vi "Build XY Plot Histogram (Core).vi"(4 "Bin Size (Dialog)":dbl=nan, 5 "Align Histogram Bin":bool, 6 "Plot Index":i32, 7 "Max Number of Bins":i32, 8 "error in (no error)":errorcluster, 9 "Data Axis (Y: F)":bool, 10 "Mouse Click Coords":T1, 11 "XYGraph in":T2) -> (0 "error out":errorcluster, 1 "Message":string, 3 "Data Statistics":dbl[](array[numeric]))   [LabVIEW 2019, in "Histogram Window.lvlib"]
uses:
  Histogram Window.lvlib
  Graphs/XY Graph/XY Graph Refnum.ctl
  <vilib>/Utility/miscctls.llb/LVPoint32TypeDef.ctl
  Linear Histogram Options.ctl
  Histogram Bin Position.ctl
  Plot Histogram.ctl
  Graphs/Plot Style 3.ctl
  Histogram Window Q Element v2.ctl
  Histogram Window Q Action v2.ctl
  Data Statistics.ctl
  48084c95-8393-4bd0-bb26-e53c6117abf8.vi/ae578a56-f3ce-4ec2-8f3b-219cc1dae63b.vi
  <vilib>/Analysis/NI_AALBase.lvlib
  <vilib>/Analysis/NI_AALPro.lvlib
  Graphs/XY Graph/XY Graph Add-Ons.lvlib
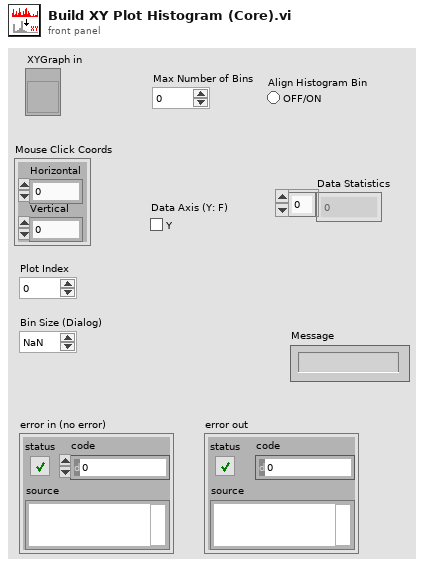
[diagram p1: front panel]
types:
  T1 = typedef "LVPoint32TypeDef.ctl" = cluster{"Horizontal":i32, "Vertical":i32}
  T2 = typedef "XY Graph Add-Ons.lvlib/XY Graph Refnum.ctl" = refnum<vi>
  T3 = typedef "Plot Style 3.ctl" = cluster{"Plot Style":enum16{"unchanged", "Line", "Symbol", "Line + Symbol", "Histogram", "Histogram + Symbol"}, "Histogram Type":enum16{"unchanged", "Left Bound", "Center", "Right Bound"}, "Line Tickness":enum16{"unchanged", "Thin", "1 pixel", "2 pixel", "3 pixel", "4 pixel", "5 pixel"}, "Line Style":enum16{"unchanged", "Plain", "Long Dash", "Short Dash", "Long-Short Dash", "Long-Short-Short Dash"}, "Point Style":enum16{"unchanged", "None", "Empty Circle", "Filled Circle", "Thick Circle", "Dotted Circle", "Empty Square", "Filled Square", "Thick Square", "Dotted Square", "Small Filled Square", "Dot", "Cross", "Tiny Cross", "Large X", "Small x", "Diamond", "Small Empty Square"}, "Line Color":u32, "Point Color":u32, "Anti-aliased":bool, "Line Color Chooser":enum16{"unchanged", "Color Box", "Color List"}, "Point Color Chooser":enum16{"unchanged", "Color Box", "Color List"}, "Line Color List":string, "Point Color List":string}
  T4 = typedef "Histogram Window.lvlib/Data Statistics.ctl" = cluster{"mean":dbl, "standard deviation":dbl, "variance":dbl, "rms value":dbl, "median":dbl, "mode":dbl, "max Value":dbl, "min Value":dbl, "# elements  ":dbl}
  T5 = typedef "Histogram Window.lvlib/Histogram Window Q Element v2.ctl" = cluster{"Histogram Window Q Action":T6, "Data":variant}
  T6 = typedef "Histogram Window.lvlib/Histogram Window Q Action v2.ctl" = enum16{"Idle", "Initialization", "Generic XY Graph Event", "Add Histogram", "Delete Plot", "Delete Selected Plots", "Clear Graph", "Change Bin Size", "Invert Histogram", "Update Graph", "Plot Fit", "Export XYGraph to Notebook", "Quit"}
  T7 = typedef "Histogram Window.lvlib/Plot Histogram.ctl" = cluster{"Plot Name":string, "Histogram":cluster{"Axis":dbl[], "Histogram":dbl[]}, "Plot Style":T3}
  T8 = typedef "Linear Histogram Options.ctl" = cluster{"Bin Size":dbl, "Min Value":dbl, "Max Value":dbl, "Filter NaN & Infinite Values":bool, "Frequency Plot":bool, "Align Bins":bool, "Bin Location":T9, "Project Outside Values":bool, "Max Histogram Size":i32}
  T9 = typedef "Histogram Bin Position.ctl" = enum16{"Left", "Center", "Right"}
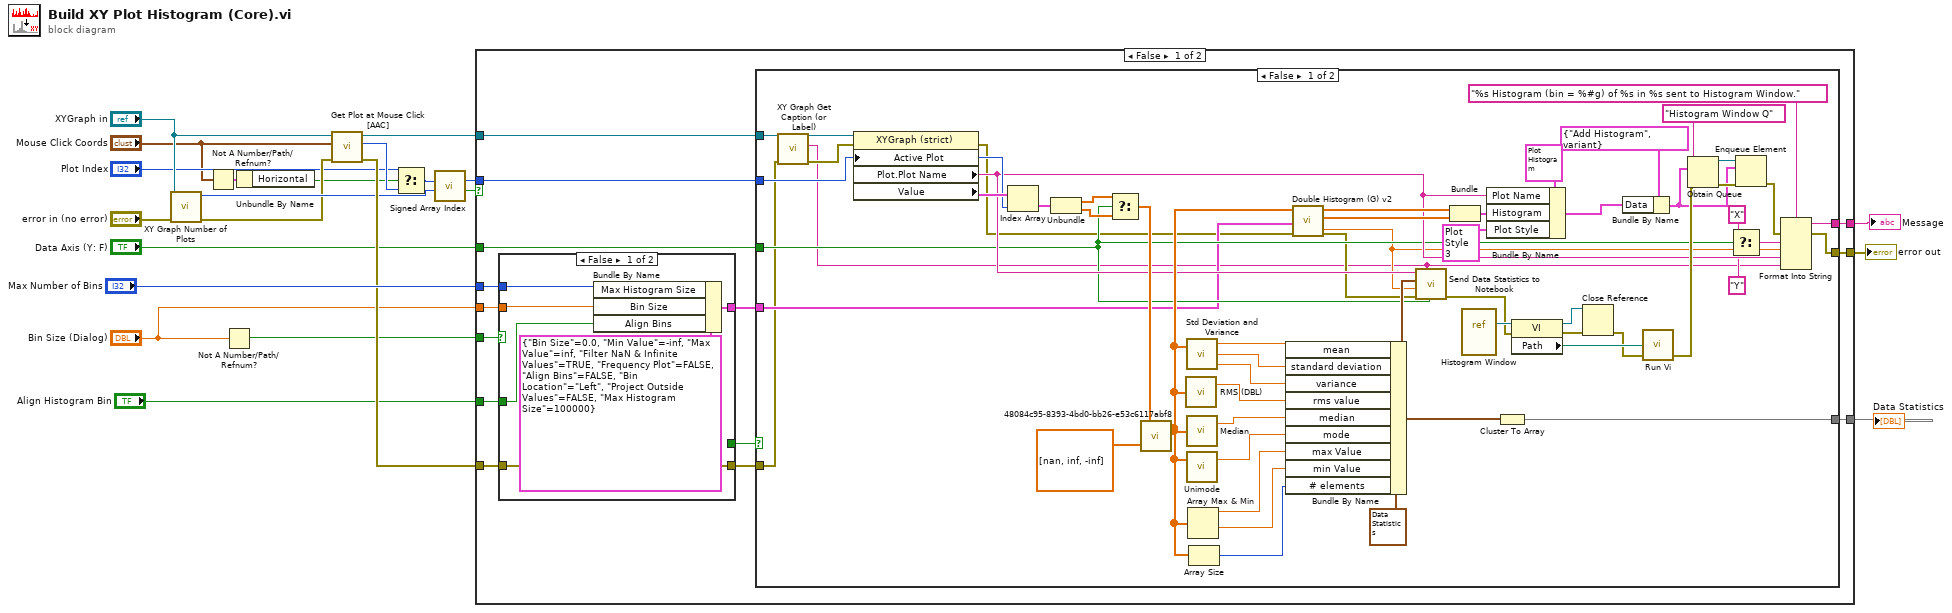
[diagram p0: block diagram]
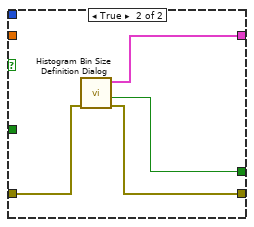
[diagram p3: hidden frame]
diagram:
  n1 = call "XY Graph Number of Plots.vi"("Error In"="error in (no error)", "XYGraph in"="XYGraph in") -> ("Error Out"=w15:errorcluster, "# Plots"=w18:i32)  [unwired: 8 in]
  n2 = Not A Number/Path/Refnum?(number/path/refnum="Mouse Click Coords") -> (NaN/Path/Refnum?=w7:cluster{"Horizontal":bool, "Vertical":bool})
  n3 = Not A Number/Path/Refnum?(number/path/refnum="Bin Size (Dialog)") -> (NaN/Path/Refnum?=w11:bool)
  n4 = Unbundle By Name(w7) -> ("Horizontal"=w8:bool)
  n5 = call "Get Plot at Mouse Click [AAC].vi"("error in (no error)"=w15, "Mouse Click Coordinates"="Mouse Click Coords", "XYGraph Ref"="XYGraph in") -> ("error out"=w20:errorcluster, "Plot at Coordinates"=w10:i32, "XYGraph Ref"=w4:T2)  [unwired: 2 in, 4 out]
  n6 = Select(t="Plot Index", s=w8, f=w10) -> (s? t:f=w16:i32)
  n7 = call "Signed Array Index.vi"("Array Size"=w18, "Array Index in"=w16) -> ("Out of Range?"=w19:bool, "Array Index out"=w17:i32)  [unwired: 8 in]
  n8 = case shown="False" w19 {
    tunnel: [w35 w104] -> w22
    tunnel: w4 -> [w36 _]
    tunnel: "Max Number of Bins" -> [w25 _]
    tunnel: w20 -> [w31 w104]
    tunnel: [w30 _] -> w5
    tunnel: w11 -> [w29 _]
    tunnel: "Bin Size (Dialog)" -> [w28 _]
    tunnel: w17 -> [w34 _]
    tunnel: "Data Axis (Y: F)" -> [w27 _]
    tunnel: [w26 _] -> w2
    tunnel: "Align Histogram Bin" -> [w23 _]
    frame False {
      n9 = case shown="False" w29 {
        tunnel: [_ w101] -> w33
        tunnel: [w99 w103] -> w32
        tunnel: w31 -> [w99 w102]
        tunnel: w28 -> [w97 _]
        tunnel: w25 -> [w98 _]
        tunnel: [w95 w100] -> w24
        tunnel: w23 -> [w94 _]
        frame False {
          n10 = Bundle By Name(cluster=T8 {"Bin Size"=0.0, "Min Value"=-inf, "Max Value"=inf, "Filter NaN & Infinite Values"=TRUE, "Frequency Plot"=FALSE, "Align Bins"=FALSE, "Bin Location"=enum."Left", "Project Outside Values"=FALSE, "Max Histogram Size"=100000} ("input cluster"), "Max Histogram Size"=w98, "Bin Size"=w97, "Align Bins"=w94) -> (w95:T8)
        }
        frame True {
          n11 = call "Histogram Bin Size Definition Dialog.vi"("error in (no error)"=w102) -> ("error out"=w103:errorcluster, "Cancelled?"=w101:bool, "Histogram Options"=w100:T8)  [unwired: 8 in]
        }
      }
      n12 = case shown="False" w33 {
        tunnel: w36 -> [w41 _]
        tunnel: [w58 w93] -> w35
        tunnel: w34 -> [w71 _]
        tunnel: w32 -> [w38 w93]
        tunnel: [w65 _] -> w30
        tunnel: w27 -> [w52 _]
        tunnel: [w57 _] -> w26
        tunnel: w24 -> [w44 _]
        frame False {
          n13 = call "XY Graph Get Caption (or Label).vi"("error in (no error)"=w38, "XYGraph in"=w41) -> ("error out"=w39:errorcluster, "Caption (or Label) Text"=w37:string, "XYGraph out"=w40:T2)  [unwired: 7 in]
          n14 = property class="XYGraph (strict)"(reference=w40, error in=w39, "Active Plot"=w71) -> (error out=w43:errorcluster, "Plot.Plot Name"=w55:string, "Value"=w84:cluster{"X Array":dbl[], "Y Array":dbl[]}[])  [unwired: 1 out]
          n15 = Index Array(array=w84, index=w71) -> (element=w83:cluster{"X Array":dbl[], "Y Array":dbl[]})
          n16 = Unbundle(w83) -> ("X Array"=w62:dbl[], "Y Array"=w61:dbl[])
          n17 = Select(t=w62, s=w52, f=w61) -> (s? t:f=w60:dbl[])
          n18 = call "48084c95-8393-4bd0-bb26-e53c6117abf8.vi"("Element(s) to Remove"=dbl[] [nan, inf, -inf], "Input Array"=w60) -> ("Output Array"=w63:dbl[])  [unwired: 1 out]
          n19 = call <vilib>:"RMS (DBL).vi"("X"=w63) -> ("rms value"=w77:dbl)  [unwired: 1 out]
          n20 = call <vilib>:"Std Deviation and Variance.vi"("X"=w63) -> ("mean"=w80:dbl, "standard deviation"=w79:dbl, "variance"=w78:dbl)  [unwired: 1 in]
          n21 = call <vilib>:"Median.vi"("X"=w63) -> ("median"=w76:dbl)  [unwired: 1 out]
          n22 = call <vilib>:"Unimode.vi"("X"=w63) -> ("mode"=w75:dbl)  [unwired: 1 in, 1 out]
          n23 = Array Max & Min(array=w63) -> (max value=w74:dbl, min value=w73:dbl)  [unwired: 2 out]
          n24 = Array Size(array=w63) -> (size(s)=w72:i32)
          n25 = Bundle By Name(cluster=T4 {"mean"=0.0, "standard deviation"=0.0, "variance"=0.0, "rms value"=0.0, "median"=0.0, "mode"=0.0, "max Value"=0.0, "min Value"=0.0, "# elements  "=0.0} ("Data Statistics"), "mean"=w80, "standard deviation"=w79, "variance"=w78, "rms value"=w77, "median"=w76, "mode"=w75, "max Value"=w74, "min Value"=w73, "# elements"=w72) -> (w66:T4)
          n26 = call "Double Histogram (G) v2.vi"("Error In"=w43, "Histogram Options"=w44, "Array"=w63) -> ("Error Out"=w42:errorcluster, "Histogram"=w86:dbl[], "Axis"=w85:dbl[], "Actual Bin Size"=w45:dbl)  [unwired: 4 in, 1 out]
          n27 = call "Send Data Statistics to Notebook.vi"("Data Axis (Y: F)"=w52, "Graph Caption"=w37, "Error In"=w42, "Bin"=w45, "Data Statistics"=w66, "Plot Name"=w55) -> ("Error Out"=w67:errorcluster)  [unwired: 5 in]
          n28 = Bundle("Axis"=w85, "Histogram"=w86) -> (w91:cluster{"Axis":dbl[], "Histogram":dbl[]})  [unwired: 1 in]
          n29 = vi-ref "Histogram Window.vi"() -> (w70:refnum<vi>)
          n30 = Bundle By Name(cluster=T7 {"Plot Name"="", "Histogram"={"Axis"=[], "Histogram"=[]}, "Plot Style"={"Plot Style"=enum."Histogram + Symbol", "Histogram Type"=enum."Right Bound", "Line Tickness"=enum."unchanged", "Line Style"=enum."unchanged", "Point Style"=enum."unchanged", "Line Color"=0, "Point Color"=0, "Anti-aliased"=FALSE, "Line Color Chooser"=enum."unchanged", "Point Color Chooser"=enum."unchanged", "Line Color List"="", "Point Color List"=""}} ("output cluster"), "Plot Name"=w55, "Histogram"=w91, "Plot Style"=T3 {"Plot Style"=enum."Histogram", "Histogram Type"=enum."Left Bound", "Line Tickness"=enum."1 pixel", "Line Style"=enum."Plain", "Point Style"=enum."None", "Line Color"=0, "Point Color"=0, "Anti-aliased"=TRUE, "Line Color Chooser"=enum."Color Box", "Point Color Chooser"=enum."unchanged", "Line Color List"="", "Point Color List"=""}) -> (w87:T7)
          n31 = Cluster To Array(cluster=w66) -> (array=w65:dbl[])
          n32 = property class="VI"(reference=w70, error in=w67) -> (reference out=w69:refnum<vi>, error out=w47:errorcluster, "Path"=w68:path)
          n33 = Close Reference(reference=w69, error in (no error)=w47) -> (error out=w46:errorcluster)
          n34 = Bundle By Name(cluster=T5 {"Histogram Window Q Action"=enum."Add Histogram", "Data"=variant} ("ALEX TT Histogram Q Element"), "Data"=w87) -> (w53:T5)
          n35 = call "Run Vi.vi"("VI Path"=w68, "error in (no error)"=w46) -> ("error out"=w82:errorcluster)  [unwired: 6 in, 1 out]
          n36 = Obtain Queue(name (unnamed)="Histogram Window Q", element data type=w53, error in (no error)=w82) -> (queue out=w90:refnum<queue>, error out=w88:errorcluster)  [unwired: 2 in, 1 out]
          n37 = Select(t="X" ("input 1"), s=w52, f="Y" ("input 1")) -> (s? t:f=w51:string)
          n38 = Enqueue Element(queue=w90, element=w53, error in (no error)=w88) -> (error out=w59:errorcluster)  [unwired: 1 in, 2 out]
          n39 = Format Into String(format string="%s Histogram (bin = %#g) of %s in %s sent to Histogram Window.", error in=w59, w51, w45, w55, w37) -> (resulting string=w57:string, error out=w58:errorcluster)  [unwired: 1 in]
        }
        frame True {
        }
      }
    }
    frame True {
    }
  }
  "error out" <- w22
  "Data Statistics" <- w5
  "Message" <- w2
